vi "LV XML Text Replace.vi"(8 "Text":string, 9 "Tag":string, 10 "Datatype":string, 11 "LV XML in":string) -> (3 "LV XML out":string)   [LabVIEW 2021, in "BS120x Driver.lvlib" / "ENET_BS1200.lvclass"]
uses:
  ENET_BS1200.lvclass
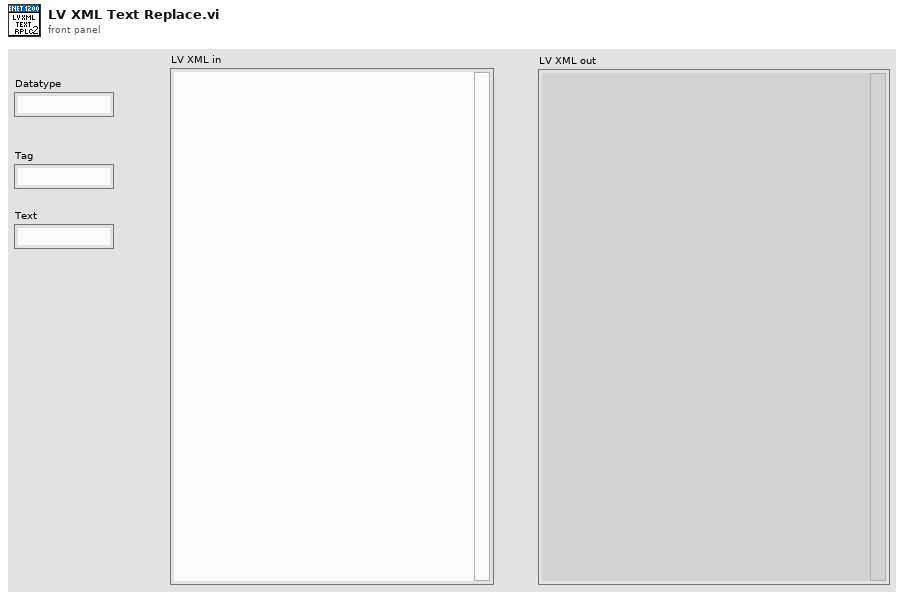
[diagram p1: front panel]
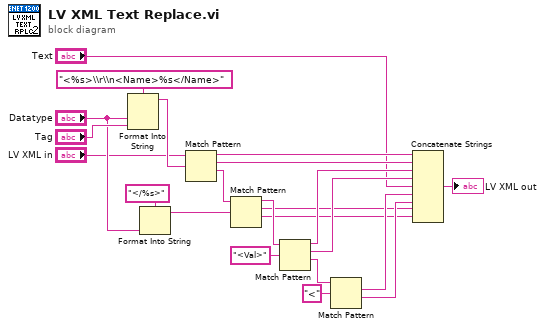
[diagram p0: block diagram]
diagram:
  n1 = Format Into String(format string="<%s>\\r\\n<Name>%s</Name>", "Datatype", "Tag") -> (resulting string=w20:string)  [unwired: 2 in, 1 out]
  n2 = Format Into String(format string="</%s>", "Datatype") -> (resulting string=w17:string)  [unwired: 2 in, 1 out]
  n3 = Match Pattern(string="LV XML in", regular expression=w20) -> (before substring=w13:string, match substring=w12:string, after substring=w11:string)  [unwired: 1 in, 1 out]
  n4 = Match Pattern(string=w11, regular expression=w17) -> (before substring=w10:string, match substring=w4:string, after substring=w3:string)  [unwired: 1 in, 1 out]
  n5 = Match Pattern(string=w10, regular expression="<Val>") -> (before substring=w9:string, match substring=w8:string, after substring=w15:string)  [unwired: 1 in, 1 out]
  n6 = Match Pattern(string=w15, regular expression="<") -> (match substring=w6:string, after substring=w5:string)  [unwired: 1 in, 2 out]
  n7 = Concatenate Strings(w13, w12, w9, w8, "Text", w6, w5, w4, w3) -> (→"LV XML out":string)
